vi "Result_Test.vi"(8 "error in (no error)":errorcluster caption="entrée d'erreur (pas d'erreur)", 11 "Get_Voltage en entrée":refnum<class "Close_Instr.lvclass">) -> (0 "error out":errorcluster caption="sortie d'erreur", 3 "Get_Voltage en sortie":refnum<class "Close_Instr.lvclass">)   [LabVIEW 2020, in "Library Test.lvlib" / "Close_Instr.lvclass"]
uses:
  Close_Instr.lvclass
  C:/Users/ngarcin/OneDrive - Altyor/Standard TB/Class/Test/Test (Default)/Test (Default).lvclass
  Test_Wtih_Instr/Test_With_Inst.lvclass
  Close_Instr.lvclass/Close_Instr.ctl
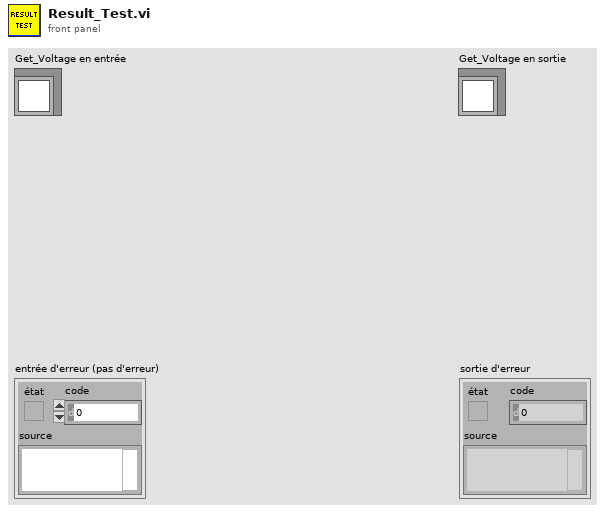
[diagram p1: front panel]
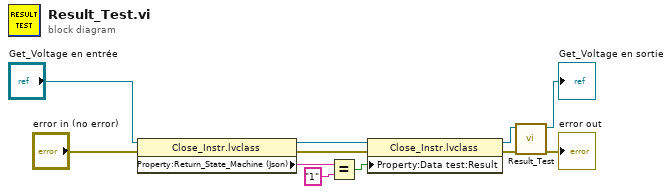
[diagram p0: block diagram]
diagram:
  n1 = property class="Close_Instr.lvclass"(reference="Get_Voltage en entrée", error in="error in (no error)") -> (reference out=w8:refnum<class "Close_Instr.lvclass">, error out=w7:errorcluster, "Property:Return_State_Machine (Json)"=w3:string)
  n2 = Equal?(x=w3, y="1") -> (x = y?=w1:bool)
  n3 = property class="Close_Instr.lvclass"(reference=w8, error in=w7, "Property:Data test:Result"=w1) -> (reference out=w4:refnum<class "Close_Instr.lvclass">, error out=w5:errorcluster)
  n4 = call-parent "Result_Test.vi"("error in (no error)"=w5, "Test_With_Inst en entrée"=w4) -> ("error out"=→"error out":errorcluster, "Test_With_Inst en sortie"=→"Get_Voltage en sortie":refnum<class "Close_Instr.lvclass">)  [unwired: 8 in]
